vi "Rotate.vi"(8 "error in (no error)":errorcluster, 10 "Angle (deg)":dbl, 11 "Image in":refnum<class "Image.lvclass">) -> (0 "error out":errorcluster, 3 "Image out":refnum<class "Image.lvclass">)   [LabVIEW 2021, in "Picture2D.lvlib" / "Image.lvclass"]
uses:
  Image.lvclass
  Image.lvclass/Image.ctl
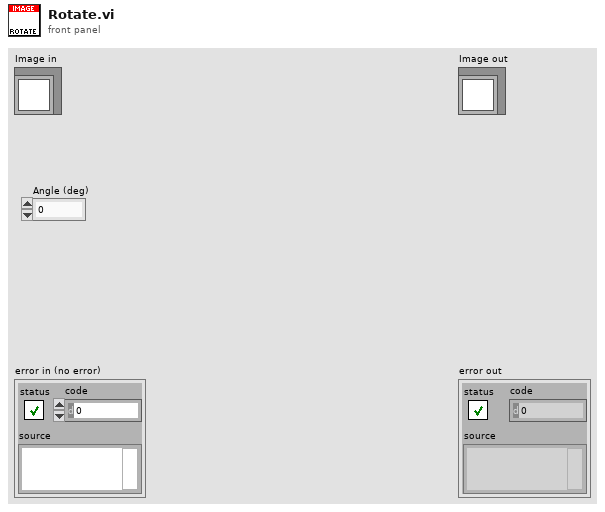
[diagram p1: front panel]
types:
  T1 = typedef "imagedata.ctl" = cluster{"image type":i32, "image depth":i32, "image":u8[], "mask":u8[], "colors":u32[], "Rectangle":cluster{"left":i16, "top":i16, "right":i16, "bottom":i16}}
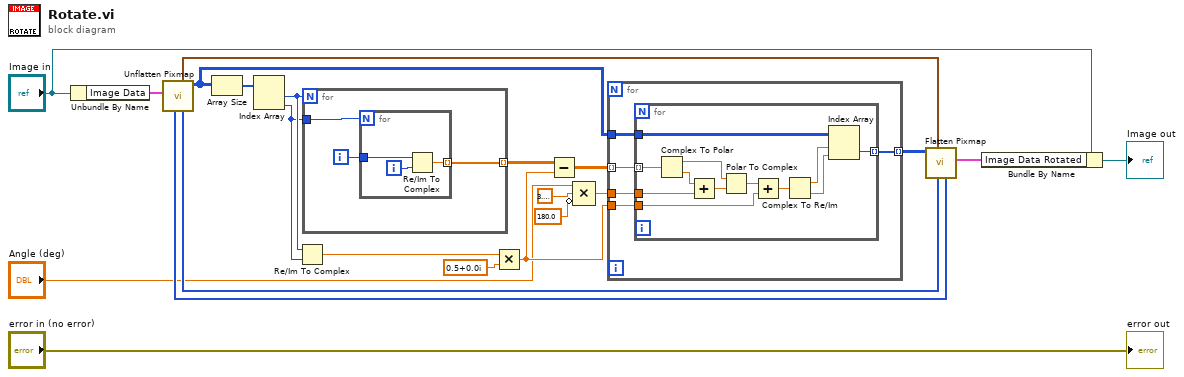
[diagram p0: block diagram]
diagram:
  n1 = Unbundle By Name("Image in") -> ("Image Data"=w21:T1)
  n2 = call <vilib>:"Unflatten Pixmap.vi"("image data"=w21) -> ("24-bit pixmap"=w10:u32[][], "colors"=w6:u32[], "top left"=w7:cluster{"x":i16, "y":i16}, "mask"=w5:u8[])  [unwired: 4 in, 3 out]
  n3 = Array Size(array=w10) -> (size(s)=w20:i32[])
  n4 = Index Array(array=w20) -> (element #1=w16:i32, element #2=w15:i32)  [unwired: 2 in]
  n5 = Re/Im To Complex(1:w15, 2:w16) -> (0:w19:cdb)
  n6 = for {
    N: w16 -> [_]
    tunnel: [w24] -> w17 mode=indexing
    tunnel: w15 -> [w23]
    i -> [w25]
    n7 = for {
      N: w23 -> [_]
      tunnel: w25 -> [w27]
      tunnel: [w26] -> w24 mode=indexing
      i -> [w28]
      n8 = Re/Im To Complex(1:w28, 2:w27) -> (0:w26:cdb)
    }
  }
  n9 = Multiply(x=w19, y=cdb 0.5+0.0i) -> (x*y=w11:cdb)
  n10 = Subtract(x=w17, y=w11) -> (x-y=w9:cdb[][])
  n11 = Compound Arithmetic op=MULTIPLY("Angle (deg)", 3.141592653589793, invert 180.0 ("value")) -> (w12:dbl)
  n12 = for {
    tunnel: w12 -> [w33]
    tunnel: w11 -> [w32]
    tunnel: w10 -> [w31]
    tunnel: w9 -> [w30] mode=indexing
    tunnel: [w29] -> w8 mode=indexing
    n13 = for {
      tunnel: w31 -> [w40]
      tunnel: w33 -> [w42]
      tunnel: w32 -> [w37]
      tunnel: w30 -> [w36] mode=indexing
      tunnel: [w35] -> w29 mode=indexing
      n14 = Complex To Polar(r * e^(i*theta)=w36) -> (r=w45:dbl, theta=w44:dbl)
      n15 = Add(x=w44, y=w42) -> (x+y=w43:dbl)
      n16 = Polar To Complex(1:w43, 2:w45) -> (0:w41:cdb)
      n17 = Add(x=w41, y=w37) -> (x+y=w38:cdb)
      n18 = Complex To Re/Im(x + iy=w38) -> (x=w34:dbl, y=w39:dbl)
      n19 = Index Array(array=w40, index (row)=w34, index (col)=w39) -> (element=w35:u32)
    }
  }
  n20 = call <vilib>:"Flatten Pixmap.vi"("mask"=w5, "colors"=w6, "top left"=w7, "24-bit pixmap"=w8) -> ("image data"=w2:T1)  [unwired: 7 in]
  n21 = Bundle By Name(cluster="Image in", "Image Data Rotated"=w2) -> (→"Image out":refnum<class "Image.lvclass">)
  "error out" <- "error in (no error)"
